vi "TCP Read - Array of Characters.vi"(8 "error in":errorcluster, 10 "timeout ms (default 50ms)":i32=50, 11 "TCP Network Connection in":refnum<k5>) -> (0 "error out":errorcluster, 2 "Characters Read":string[](array[string]), 3 "TCP Network Connection out":refnum<k5>)   [LabVIEW 2017, in "Communications Library.lvlib"]
doc: "Reads characters one by one from the TCP port.\nExits, when a new character has not been read within the timeout time."
uses:
  Communications Library.lvlib
  Error 5102 - DTACQ unit replied with an error--const.vi
  <vilib>/Utility/error.llb/Error Cluster From Error Code.vi
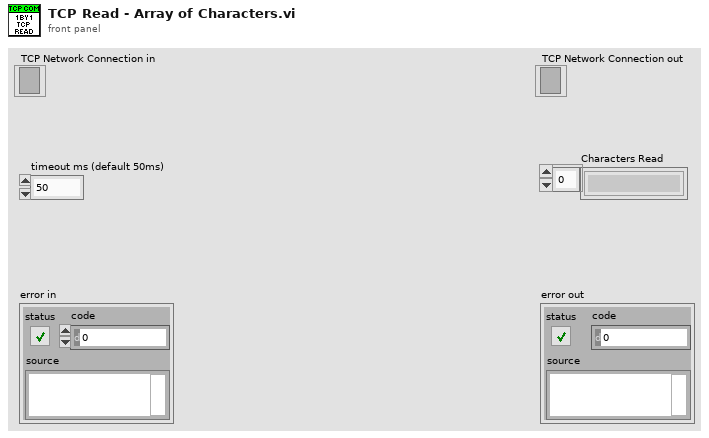
[diagram p1: front panel]
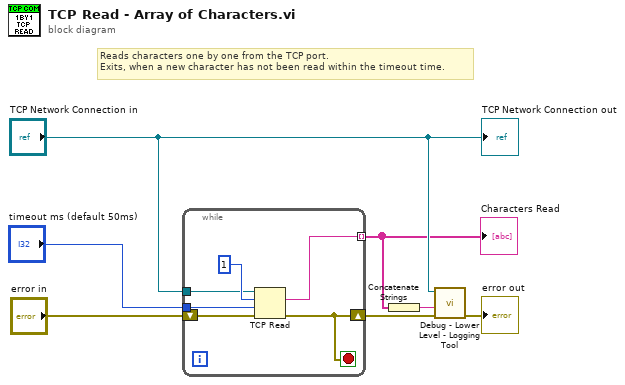
[diagram p0: block diagram]
diagram:
  # "Reads characters one by one from the TCP port.\nExits, when a new character has not been read within the timeout time."
  n1 = while {
    tunnel: [w13] -> w2 mode=indexing
    shift-right: [w10] -> w5
    shift-left: "error in" -> [w12]
    tunnel: "timeout ms (default 50ms)" -> [w9]
    tunnel: "TCP Network Connection in" -> [w8]
    stop <- w10 stop-if-true
    n2 = TCP Read(connection ID=w8, bytes to read=1, error in (no error)=w12, 9:w9) -> (data out=w13:string, error out=w10:errorcluster)  [unwired: 1 in, 1 out]
  }
  "Characters Read" <- w2
  n3 = Concatenate Strings(w2) -> (w1:string)
  n4 = call "Debug - Lower Level - Logging Tool.vi"("Error In"=w5, "Data Received"=w1, "TCP Network Connecion In"="TCP Network Connection in") -> ("Error Out"=→"error out":errorcluster)  [unwired: 7 in, 1 out]
  "TCP Network Connection out" <- "TCP Network Connection in"
